vi "DDS_ramp.vi"() -> ()   [LabVIEW 2017]
uses:
  <vilib>/eio/EIONode/EIONode.xnode
  <vilib>/rvi/eio/common/nirviEmuTemplateMethod_errors.vi
  <vilib>/Platform/TimedLoop/XDataNode/XDataNode.xnode
  <vilib>/Platform/TimedLoop/XDataNode/nitl_modes.ctl
  <vilib>/Platform/TimedLoop/XDataNode/XDNodeRunTimeDep.lvlib
  <vilib>/Platform/TimedLoop/XDataNode/wakeup.ctl
  <vilib>/Platform/TimedLoop/XDataNode/timing_clust.ctl
panel:
  out "shift reg indicator":bool
  in  "Numeric":u64=50
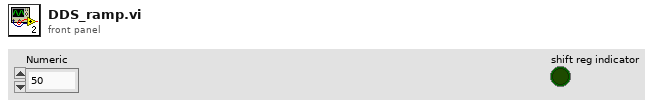
[diagram p1: front panel]
types:
  T1 = typedef "XDNodeRunTimeDep.lvlib/timing_clust.ctl" = cluster{"Expected End [f-1]":u64, "Actual End [f-1]":u64, "Finished Late? [f-1]":bool, "Expected End [i-1]":u64, "Actual End [i-1]":u64, "Finished Late? [i-1]":bool, "Expected Start [i]":u64, "Actual Start [i]":u64, "Expected Start [f]":u64, "Actual Start [f]":u64, "Source Name":string, "Structure Name":string, "Period":i64, "Deadline":i64, "Offset":i64, "Start":i64, "Priority":i32, "Timeout":i32, "Mode":T2, "Wakeup Reason":T3, "Error":errorcluster, "Source Type":string, "Secondary Source Type":string, "Global End Time":u64, "Global Start Time":u64, "Frame Duration":u64, "Iteration Duration":u64, "Assigned CPU":i32, "I/O Scan Engine Mode":u32}
  T2 = typedef "XDNodeRunTimeDep.lvlib/nitl_modes.ctl" = enum32{"No Change", "Process missed periods, maintain original phase", "Discard missed periods, maintain original phase", "Process missed periods, ignore original phase", "Discard missed periods, ignore original phase"}
  T3 = typedef "XDNodeRunTimeDep.lvlib/wakeup.ctl" = enum32{"Normal", "Aborted", "Asynchronous wakeup", "Timing source error", "Timed loop error", "Timeout"}
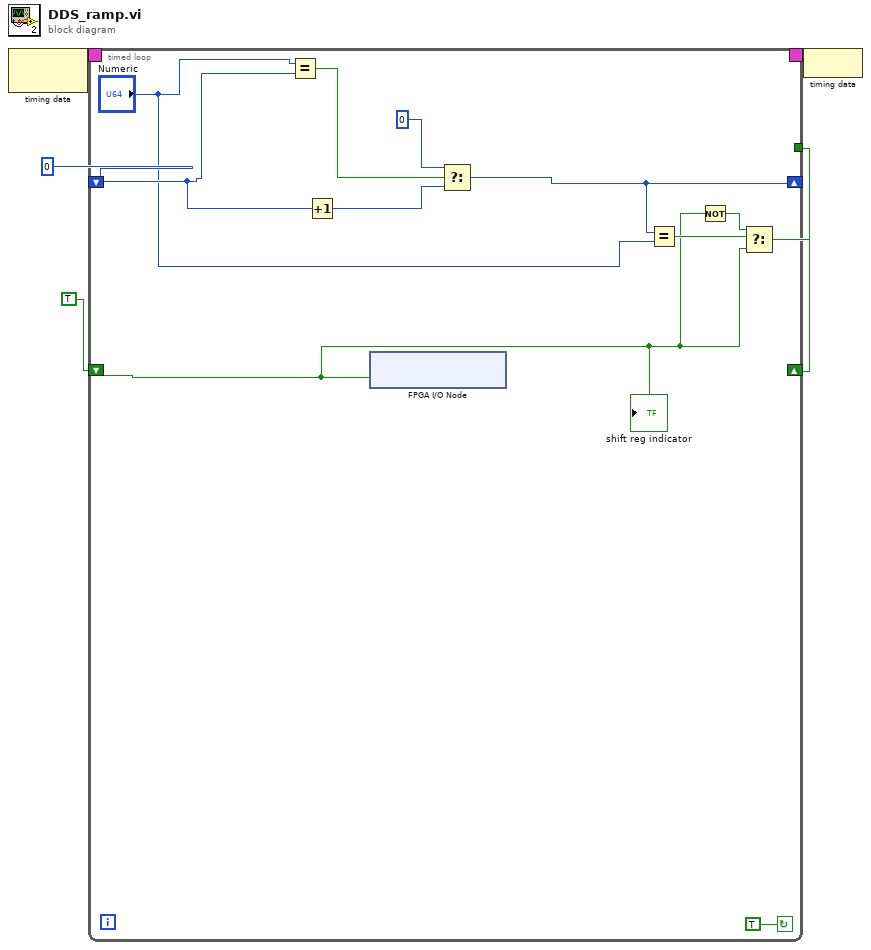
[diagram p0: block diagram]
diagram:
  n1 = node-c288() -> (w2:T1)  [unwired: 1 in]
  n2 = timed-loop {
    shift-right: [w8] -> _
    shift-left: u64 0 -> [w14]
    shift-right: [w5] -> _
    shift-left: TRUE -> [w6]
    timing: w2 -> [_]
    timing-out: [_] -> w1
    tunnel: [w5] -> _
    stop <- TRUE continue-if-true
    n3 = Equal?(x="Numeric", y=w14) -> (x = y?=w12:bool)
    n4 = Increment(x=w14) -> (x+1=w13:u64)
    n5 = xnode "FPGA I/O Node"("Connector1/DIO6"=w6) -> ()  [unwired: 1 in, 1 out]
    n6 = Select(t=i16 0, s=w12, f=w13) -> (s? t:f=w8:u64)
    n7 = Equal?(x=w8, y="Numeric") -> (x = y?=w7:bool)
    n8 = Not(x=w6) -> (.not. x?=w10:bool)
    n9 = Select(t=w10, s=w7, f=w6) -> (s? t:f=w5:bool)
    "shift reg indicator" <- w6
  }
  n10 = node-c288(w1) -> ()
